vi "Help_geral.vi"() -> ()   [LabVIEW 2019]
panel:
  in  "Array":T1(array[cluster])
  in  "[ESC]":bool
  # "HELP"
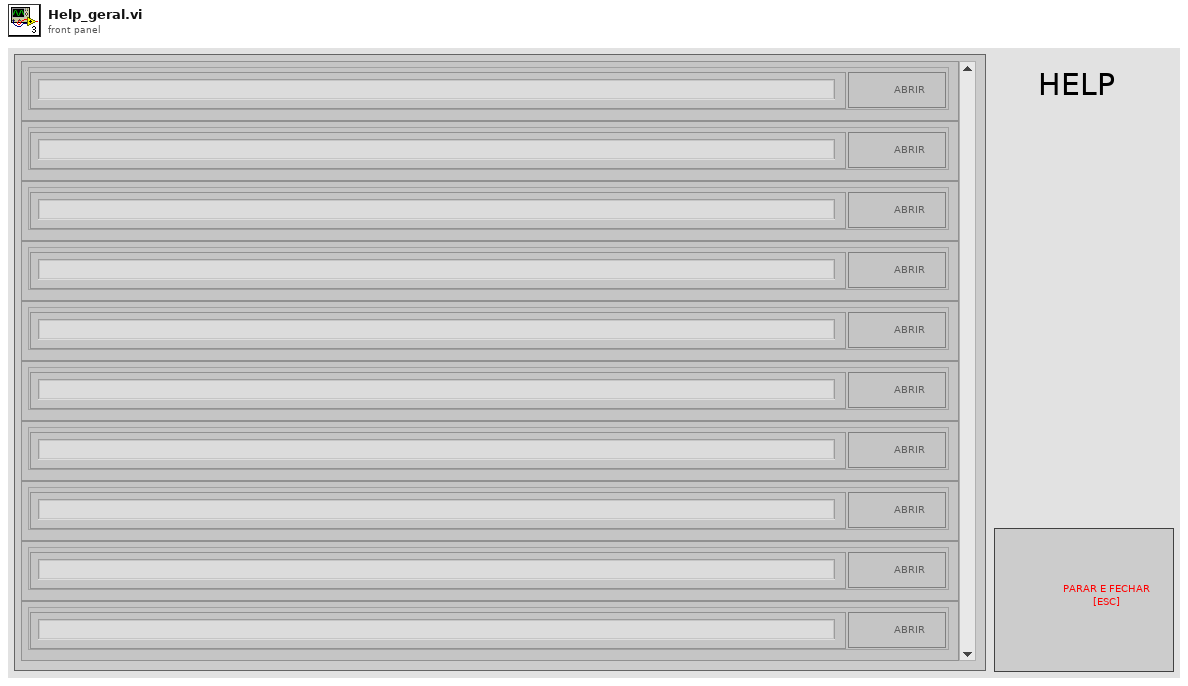
[diagram p1: front panel]
types:
  T1 = cluster{"Documento":string, "Open Button":bool}[]
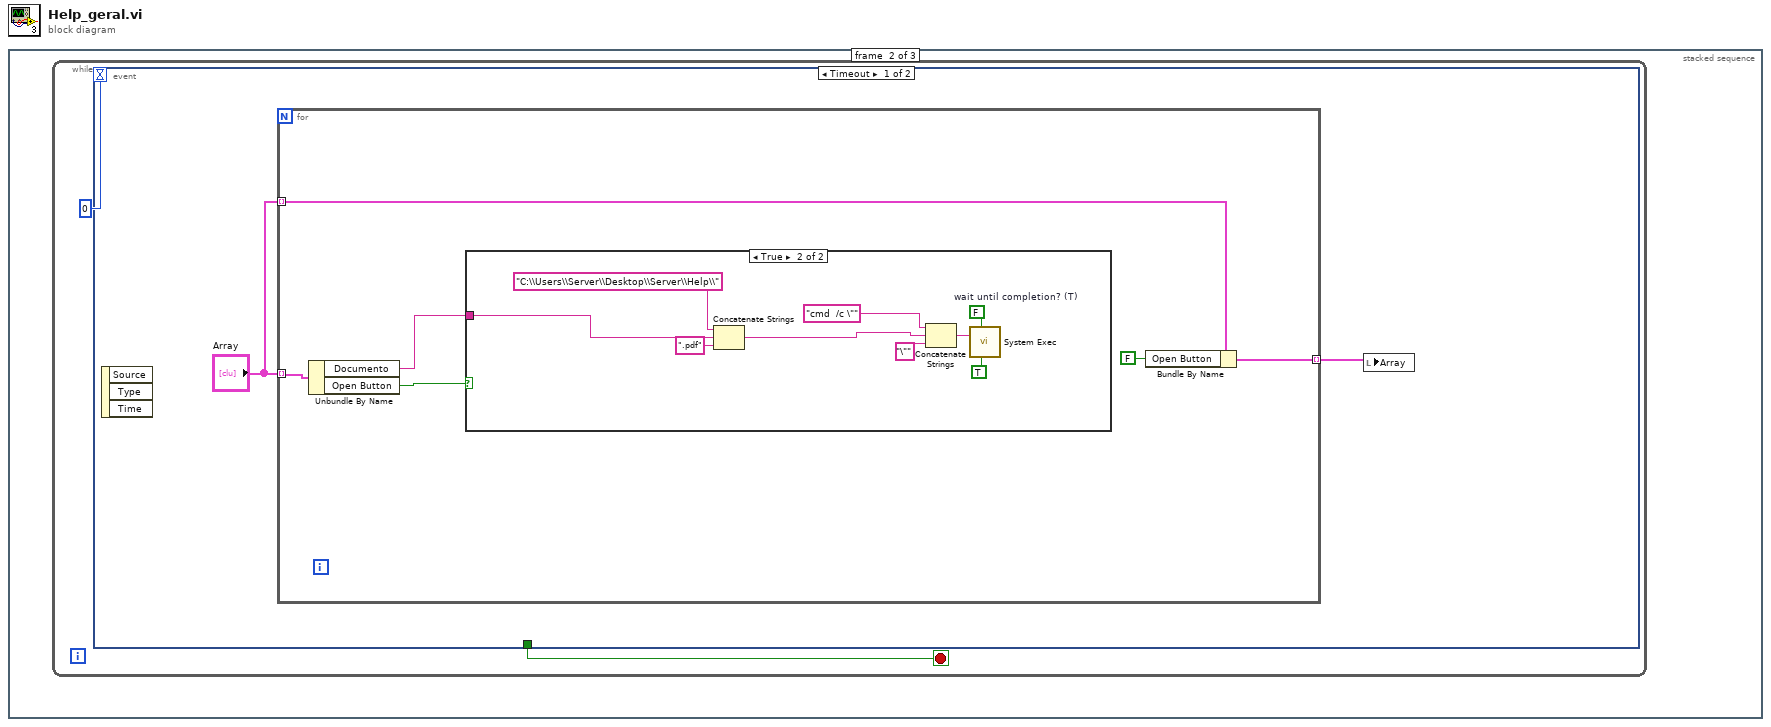
[diagram p0: block diagram]
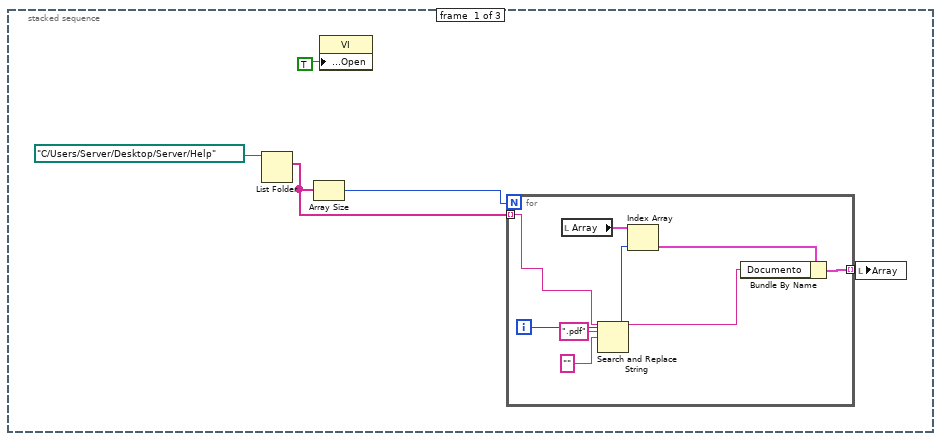
[diagram p2: hidden frame]
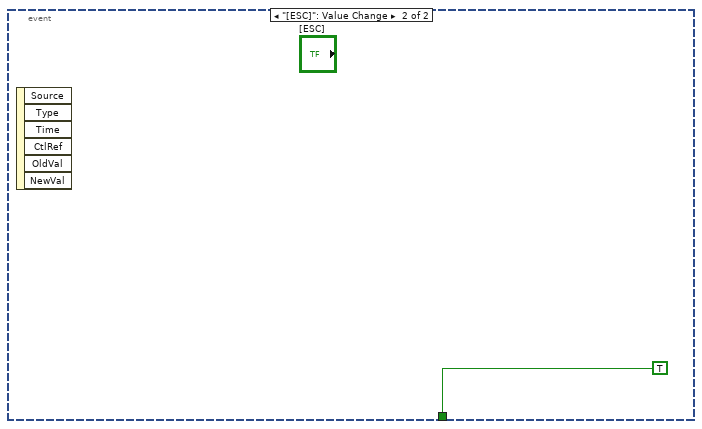
[diagram p4: hidden frame]
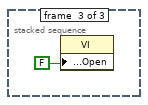
[diagram p5: hidden frame]
diagram:
  n1 = stacked-sequence {
    frame #0 {
      n2 = List Folder(path=path "C:/Users/Server/Desktop/Server/Help") -> (filenames=w3:string[])  [unwired: 3 in, 3 out]
      n3 = Array Size(array=w3) -> (size(s)=w2:i32)
      n4 = property class="VI"("Front Panel.Open"=TRUE ("Front Panel Window:Open")) -> ()  [unwired: 2 in, 2 out]
      n5 = for {
        N: w2 -> [_]
        tunnel: w3 -> [w8] mode=indexing
        tunnel: [w10] -> w1 mode=indexing
        i -> [w12]
        n6 = local read "Array"() -> (w13:T1)
        n7 = Search and Replace String(input string=w8, search string=".pdf", replace string="" ("replace string (\"\")")) -> (result string=w6:string)  [unwired: 5 in, 3 out]
        n8 = Index Array(array=w13, index=w12) -> (element=w11:cluster{"Documento":string, "Open Button":bool})
        n9 = Bundle By Name(cluster=w11, "Documento"=w6) -> (w10:cluster{"Documento":string, "Open Button":bool})
      }
      n10 = local write "Array"(w1) -> ()
    }
    frame #1 {
      n11 = while {
        stop <- w15 stop-if-true
        n12 = event shown="[0] Timeout" {
          selector: _ -> [_ _]
          dyn-events: _ -> [_ _]
          timeout: 0 -> [_ _]
          tunnel: [_ TRUE] -> w15
          event Timeout {
            n13 = event-data() -> ()  [unwired: 1 in, 3 out]
            n14 = for {
              tunnel: "Array" -> [w23] mode=indexing
              tunnel: "Array" -> [w20] mode=indexing
              tunnel: [w19] -> w16 mode=indexing
              n15 = Unbundle By Name(w23) -> ("Documento"=w21:string, "Open Button"=w22:bool)
              n16 = case shown="True" w22 {
                tunnel: w21 -> [_ w26]
                frame False {
                }
                frame True {
                  w32 = FALSE  # wait until completion? (T)
                  n17 = Concatenate Strings("C:\\Users\\Server\\Desktop\\Server\\Help\\", w26, ".pdf" ("string")) -> (w24:string)
                  n18 = Concatenate Strings("cmd  /c \"", w24, "\"") -> (w30:string)
                  n19 = call <vilib>:"System Exec.vi"("run minimized? (F)"=TRUE, "wait until completion? (T)"=w32, "command line"=w30) -> ()  [unwired: 5 in, 4 out]
                }
              }
              n20 = Bundle By Name(cluster=w20, "Open Button"=FALSE ("Abrir Certificado")) -> (w19:cluster{"Documento":string, "Open Button":bool})
            }
            n21 = local write "Array"(w16) -> ()
          }
          event "[ESC]": Value Change {
            n22 = event-data() -> ()  [unwired: 1 in, 6 out]
          }
        }
      }
    }
    frame #2 {
      n23 = property class="VI"("Front Panel.Open"=FALSE ("Front Panel Window:Open")) -> ()  [unwired: 2 in, 2 out]
    }
  }
